vi "Subvi flush memory.vi"(1 "Memory In":refnum<k21>="ABUF0tmp") -> ()   [LabVIEW 2017]
uses:
  <vilib>/rvi/DataTransferAndStorage/Container/Common/niFpgaContainerExecOnDevCompGetState.vi
  <vilib>/rvi/Emulation/niFpgaEmulationIsFPGAContextNoSignature.vi
  <vilib>/rvi/DataTransferAndStorage/Container/Common/niFpgaContainerGetUniqueNameForEmu.vi
  <vilib>/rvi/Emulation/niFpgaProcessEmulError.vi
  <vilib>/rvi/Emulation/niFpgaSctlEmulationGetInTimedLoop.vi
  <vilib>/rvi/errors/nirviReportUnexpectedCaseInternalError (U32).vi
  <vilib>/rvi/Memory/Memory_Emulation/niFpgaMemoryEmulationCacheClearOnFirstRun.vi
  <vilib>/rvi/Memory/Memory_Emulation/nirvimemoryEmulationManagerCache_MakeExclusive.vi
  <vilib>/rvi/Memory/Memory_Emulation/niFpgaMemoryEmulationValidateCache.vi
  <vilib>/rvi/Memory/Memory_Emulation/nirvimemoryEmulationManagerCache_InsertValue.vi
  <vilib>/Utility/error.llb/Clear Errors.vi
  <vilib>/rvi/Memory/Memory_Emulation/nirvimemoryEmulationManagerCache_ReleaseExclusive.vi
  <vilib>/rvi/Memory/Memory_Emulation/nirvimemoryEmulationManagerCache_GetValue.vi
  <vilib>/rvi/Memory/Memory_Emulation/nirvimemoryEmulationManagerCache_SetValue.vi
  <vilib>/rvi/Emulation/niFpgaSctlEmulationResourceMgr.vi
  <vilib>/rvi/DataTransferAndStorage/Container/XNode/niFpgaContainer.xnode
  <vilib>/rvi/Memory/Memory_Emulation/niFpgaMemoryEmulationRefIn.vi
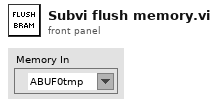
[diagram p1: front panel]
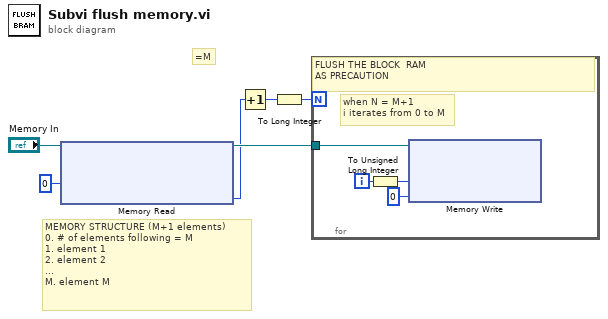
[diagram p0: block diagram]
diagram:
  # "=M"
  # "MEMORY STRUCTURE (M+1 elements)\n0. # of elements following = M\n1. element 1\n2. element 2\n...\nM. element M"
  n1 = xnode "Memory Read"("Address"=u32 0, "Memory In"="Memory In") -> ("Data"=w3:u32, "Memory Out"=w5:refnum<k21>)
  n2 = Increment(x=w3) -> (x+1=w1:u32)
  n3 = To Long Integer(number=w1) -> (32bit integer=w2:i32)
  n4 = for {
    N: w2 -> [_]
    tunnel: w5 -> [w9]
    i -> [w8]
    # "when N = M+1\ni iterates from 0 to M"
    # "FLUSH THE BLOCK  RAM\nAS PRECAUTION"
    n5 = To Unsigned Long Integer(number=w8) -> (unsigned 32bit integer=w7:u32)
    n6 = xnode "Memory Write"("Address"=w7, "Data"=u32 0, "Memory In"=w9) -> ()  [unwired: 1 out]
  }
